vi "UART 8N1 Setup.vi"(7 "Active Dut":T1, 8 "Error In":errorcluster, 10 "Baud Rate":u32, 11 "FPGA VI Reference In":refnum<k20>) -> (0 "Error Out":errorcluster, 3 "FPGA VI Reference Out":refnum<k20>)   [LabVIEW 2018]
uses:
  Resources_Test/UART/ControlTestSlot.ctl
  <vilib>/FPGAPlugInAG/PXIe-5840/niLvFpga_Run_PXIe-5840.vi
  <vilib>/Utility/error.llb/Error Cluster From Error Code.vi
  <vilib>/rvi/errors/niLvFpgaAdjustHostInterfaceError.vi
  <vilib>/rvi/interface/nirviMethod/nirviMethod.xnode
  Program Files (x86)/National Instruments/LabVIEW 2018/instr.lib/niVST/FPGA/Templates/FPGA Bitfiles/niVSTFPGA_UART.lvbitx
  <vilib>/rvi/interface/nirviReadWriteControl/nirviReadWriteControl.xnode
  NiFpgaLv.dll
  <vilib>/FPGAPlugInAG/PXIe-5840/niLvFpga_Reset_PXIe-5840.vi
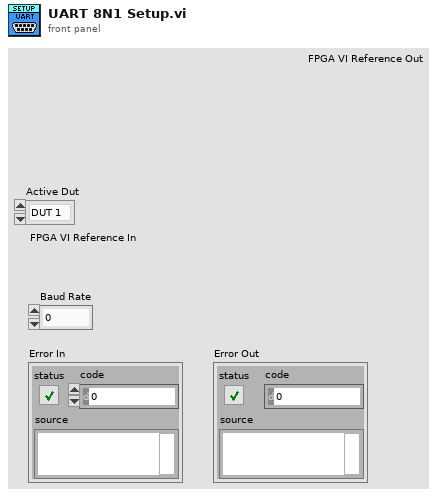
[diagram p1: front panel]
types:
  T1 = typedef "ControlTestSlot.ctl" = enum16{"DUT 1", "DUT 2"}
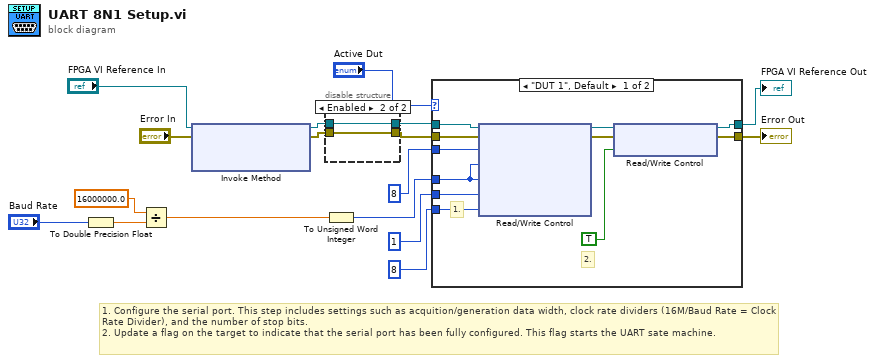
[diagram p0: block diagram]
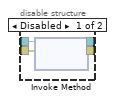
[diagram p2: hidden frame]
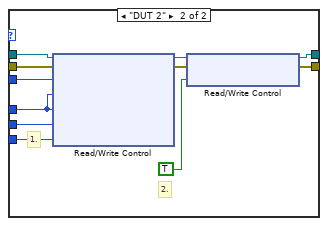
[diagram p3: hidden frame]
diagram:
  # "1. Configure the serial port. This step includes settings such as acquition/generation data width, clock rate dividers (16M/Baud Rate = Clock Rate Divider), and the number of stop bits.\n2. Update a flag on the target to indicate that the serial port has been fully configured. This flag starts the UART sate machine."
  n1 = To Double Precision Float(number="Baud Rate") -> (double precision float=w14:dbl)
  n2 = Divide(x=16000000.0, y=w14) -> (x/y=w12:dbl)
  n3 = xnode "Invoke Method"("FPGA VI Reference In"="FPGA VI Reference In", "error in"="Error In") -> ("FPGA VI Reference Out"=w4:refnum<k20>, "error out"=w3:errorcluster)  [unwired: 1 in]
  n4 = disable-structure shown="Enabled" {
    disable-tunnel: w4 -> [w21 w23]
    disable-tunnel: w3 -> [w20 w22]
    disable-tunnel: [w19 w23] -> w2
    disable-tunnel: [w18 w22] -> w1
    frame Disabled {
      n5 = xnode "Invoke Method"("FPGA VI Reference In"=w21, "error in"=w20) -> ("FPGA VI Reference Out"=w19:refnum<k20>, "error out"=w18:errorcluster)
    }
    frame Enabled {
    }
  }
  n6 = To Unsigned Word Integer(number=w12) -> (unsigned 16bit integer=w15:u16)
  n7 = case shown="\"DUT 1\", Default" "Active Dut" {
    tunnel: [w34 w45] -> w17
    tunnel: [w33 w44] -> w7
    tunnel: w1 -> [w25 w43]
    tunnel: w2 -> [w24 w42]
    tunnel: w15 -> [w29 w38]
    tunnel: u16 8 ("Acq Data Width") -> [w28 w37]
    tunnel: u16 1 ("Stop Bits") -> [w27 w36]
    tunnel: u16 8 ("Gen Data Width") -> [w26 w35]
    frame "DUT 1", Default {
      # "1."
      # "2."
      n8 = xnode "Read/Write Control"("FPGA VI Reference In"=w24, "error in"=w25, "AcqData Width"=w28, "Gen Clock Divider"=w29, "Acq Clock Divider"=w29, "Stop Bit Width"=w27, "Data Width"=w26) -> ("FPGA VI Reference Out"=w31:refnum<k20>, "error out"=w32:errorcluster)
      n9 = xnode "Read/Write Control"("FPGA VI Reference In"=w31, "error in"=w32, "Port Configured"=TRUE ("Write Data")) -> ("FPGA VI Reference Out"=w33:refnum<k20>, "error out"=w34:errorcluster)
    }
    frame "DUT 2" {
      # "1."
      # "2."
      n10 = xnode "Read/Write Control"("FPGA VI Reference In"=w42, "error in"=w43, "AcqData Width 2"=w37, "Gen Clock Divider 2"=w38, "Acq Clock Divider 2"=w38, "Stop Bit Width 2"=w36, "Data Width 2"=w35) -> ("FPGA VI Reference Out"=w40:refnum<k20>, "error out"=w41:errorcluster)
      n11 = xnode "Read/Write Control"("FPGA VI Reference In"=w40, "error in"=w41, "Port Configured 2"=TRUE ("Write Data")) -> ("FPGA VI Reference Out"=w44:refnum<k20>, "error out"=w45:errorcluster)
    }
  }
  "Error Out" <- w17
  "FPGA VI Reference Out" <- w7
